vi "setVisaName.vi"(8 "error in (no error)":errorcluster, 10 "name":string, 11 "HamegHMPSupply in":refnum<class "HamegHMPSupply.lvclass">) -> (0 "error out":errorcluster, 3 "HamegHMPSupply out":refnum<class "HamegHMPSupply.lvclass">)   [LabVIEW 2011, in "Hardware.lvlib" / "Channels.lvlib" / "HamegHMPSupply.lvclass"]
uses:
  HamegHMPSupply.lvclass
  HamegHMPSupply.lvclass/HamegHMPSupply.ctl
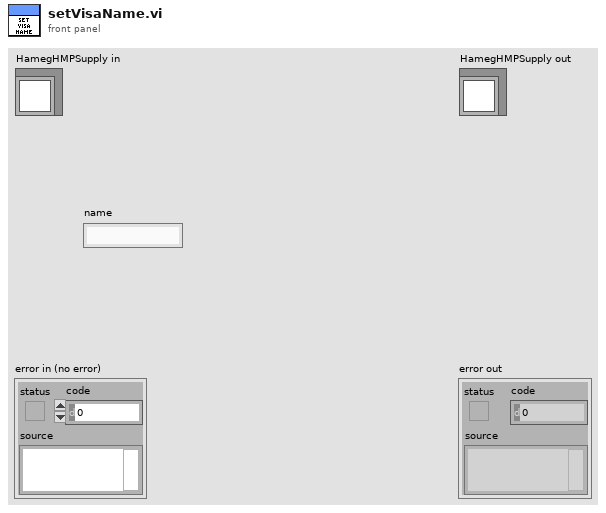
[diagram p1: front panel]
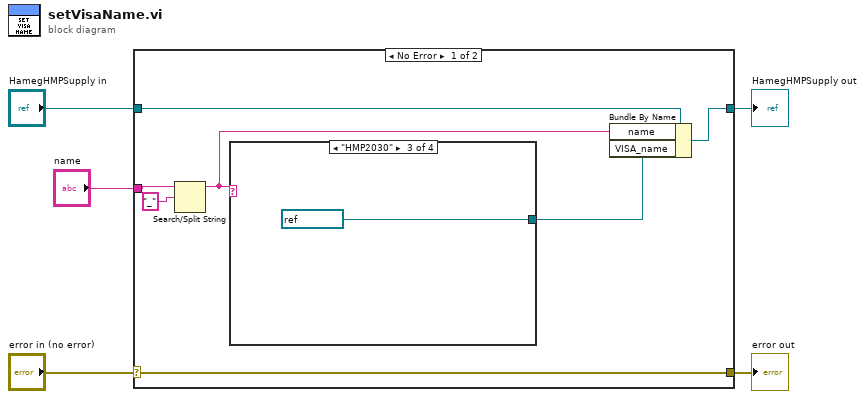
[diagram p0: block diagram]
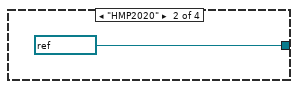
[diagram p3: hidden frame]
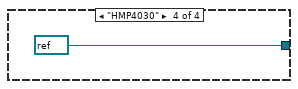
[diagram p4: hidden frame]
diagram:
  n1 = case shown="No Error" "error in (no error)" {
    selector: "error in (no error)" -> [w12 w17]
    tunnel: [w12 w17] -> w4
    tunnel: [w8 w16] -> w2
    tunnel: "HamegHMPSupply in" -> [w9 w16]
    tunnel: "name" -> [w11 _]
    frame No Error {
      n2 = Search/Split String(string=w11, search string/char (-)="_") -> (substring before match=w6:string)  [unwired: 1 in, 2 out]
      n3 = case shown="\"HMP2030\"" w6 {
        tunnel: [_ refnum<visa-resource-name> "COM3" ("VISA resource name") refnum<visa-resource-name> "COM3" ("VISA resource name") refnum<visa-resource-name> refnum ("VISA resource name")] -> w7
        frame Default {
        }
        frame "HMP2020" {
        }
        frame "HMP2030" {
        }
        frame "HMP4030" {
        }
      }
      n4 = Bundle By Name(cluster=w9, "name"=w6, "VISA_name"=w7) -> (w8:refnum<class "HamegHMPSupply.lvclass">)
    }
    frame Error {
    }
  }
  "error out" <- w4
  "HamegHMPSupply out" <- w2
